vi "Initialize FIFO_9215.vi"(8 "error in (no error)":errorcluster, 11 "FPGA Refnum Input":refnum<k20>) -> (0 "error out":errorcluster, 3 "FPGA Refnum Output":refnum<k20>)   [LabVIEW 2018]
uses:
  <vilib>/Utility/error.llb/Error Cluster From Error Code.vi
  <vilib>/rvi/errors/niLvFpgaAdjustHostInterfaceError.vi
  <vilib>/rvi/interface/nirviMethod/nirviMethod.xnode
  <vilib>/rvi/errors/niLvFpgaMergeErrorWithErrorCode.vi
  <vilib>/FPGAPlugInAG/Dynamic/niLvFpga_ReadFifo_Dynamic.vi
  <vilib>/FPGAPlugInAG/Dynamic/niLvFpga_StartFifo_Dynamic.vi
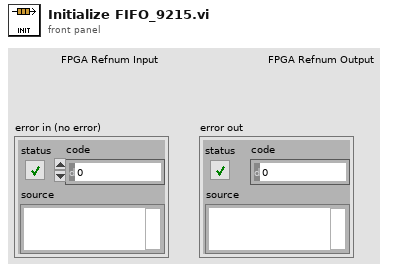
[diagram p1: front panel]
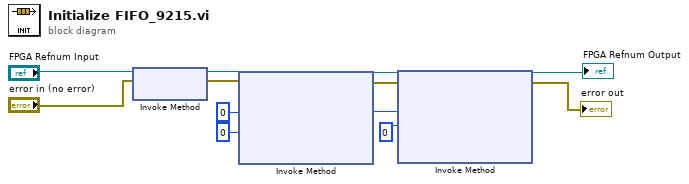
[diagram p0: block diagram]
diagram:
  n1 = xnode "Invoke Method"("FPGA VI Reference In"="FPGA Refnum Input", "error in"="error in (no error)") -> ("FPGA VI Reference Out"=w9:refnum<k20>, "error out"=w10:errorcluster)
  n2 = xnode "Invoke Method"("FPGA VI Reference In"=w9, "error in"=w10, "Number of Elements"=u32 0, "Timeout (ms)"=0) -> ("FPGA VI Reference Out"=w8:refnum<k20>, "error out"=w7:errorcluster, "Elements Remaining"=w5:u32)  [unwired: 1 out]
  n3 = xnode "Invoke Method"("FPGA VI Reference In"=w8, "error in"=w7, "Number of Elements"=w5, "Timeout (ms)"=0) -> ("FPGA VI Reference Out"=→"FPGA Refnum Output":refnum<k20>, "error out"=→"error out":errorcluster)  [unwired: 2 out]
